vi "检查前面板控件（不使用事件）.vi"() -> ()   [LabVIEW 2010]
uses:
  Instance           1 36Saved   检查前面板控件（不使用事件） .vi
panel:
  out "波形图":dynamicdata(graph)
  in  "偏置":dbl(slide)=1.3131313131313131 scale=0.0..5.0
  in  "频率":dbl(slide)=25.757575757575758 scale=0.0..50.0
  in  "幅值":dbl(slide)=5.555555555555555 scale=0.0..10.0
  in  "stop":bool
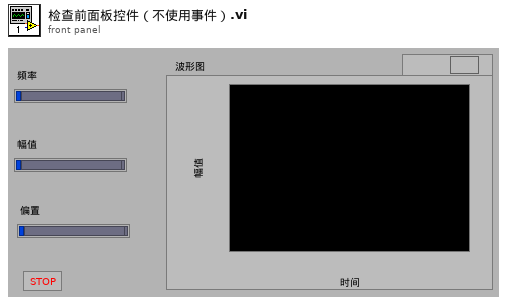
[diagram p1: front panel]
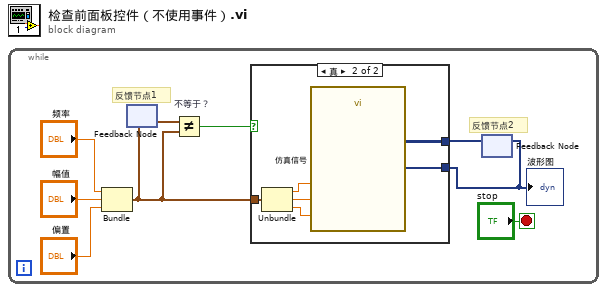
[diagram p0: block diagram]
diagram:
  n1 = while {
    stop <- "stop" stop-if-true
    # "反馈节点2"
    # "反馈节点1"
    n2 = Bundle("频率"="频率", "幅值"="幅值", "偏置"="偏置") -> (w4:cluster{"频率":dbl, "幅值":dbl, "偏置":dbl})  [unwired: 1 in]
    n3 = feedback-in #1(w4) -> ()
    n4 = feedback #1() -> (w5:cluster{"频率":dbl, "幅值":dbl, "偏置":dbl})  [unwired: 1 in]
    n5 = Not Equal? "不等于？"(x=w5, y=w4) -> (x != y?=w3:bool)
    n6 = feedback #2() -> (w2:dynamicdata)  [unwired: 1 in]
    n7 = case shown="真" w3 {
      tunnel: [w10 w15] -> w1
      tunnel: w4 -> [_ w14]
      tunnel: w2 -> [w10 _]
      frame False {
      }
      frame True {
        n8 = Unbundle(w14) -> ("频率"=w12:dbl, "幅值"=w11:dbl, "偏置"=w13:dbl)
        n9 = call "仿真信号"("Offset"=w13, "Frequency"=w12, "Amplitude"=w11) -> ("正弦"=w15:dynamicdata)  [unwired: 11 in, 1 out]
      }
    }
    "波形图" <- w1
    n10 = feedback-in #2(w1) -> ()
  }
